vi "Sam_orderfilenames.vi"(9 "Original name":string, 10 "filenames":string[](array[string])) -> (2 "Array 3":cluster{cluster{string[]}[]}[](array[cluster]))   [LabVIEW 2022 SP3]
panel:
  out "Array 2":cluster{string[]}[](array[cluster])
  out "Array":cluster{"Set":string, "Pos":i32, "hit":i32}[](array[cluster])
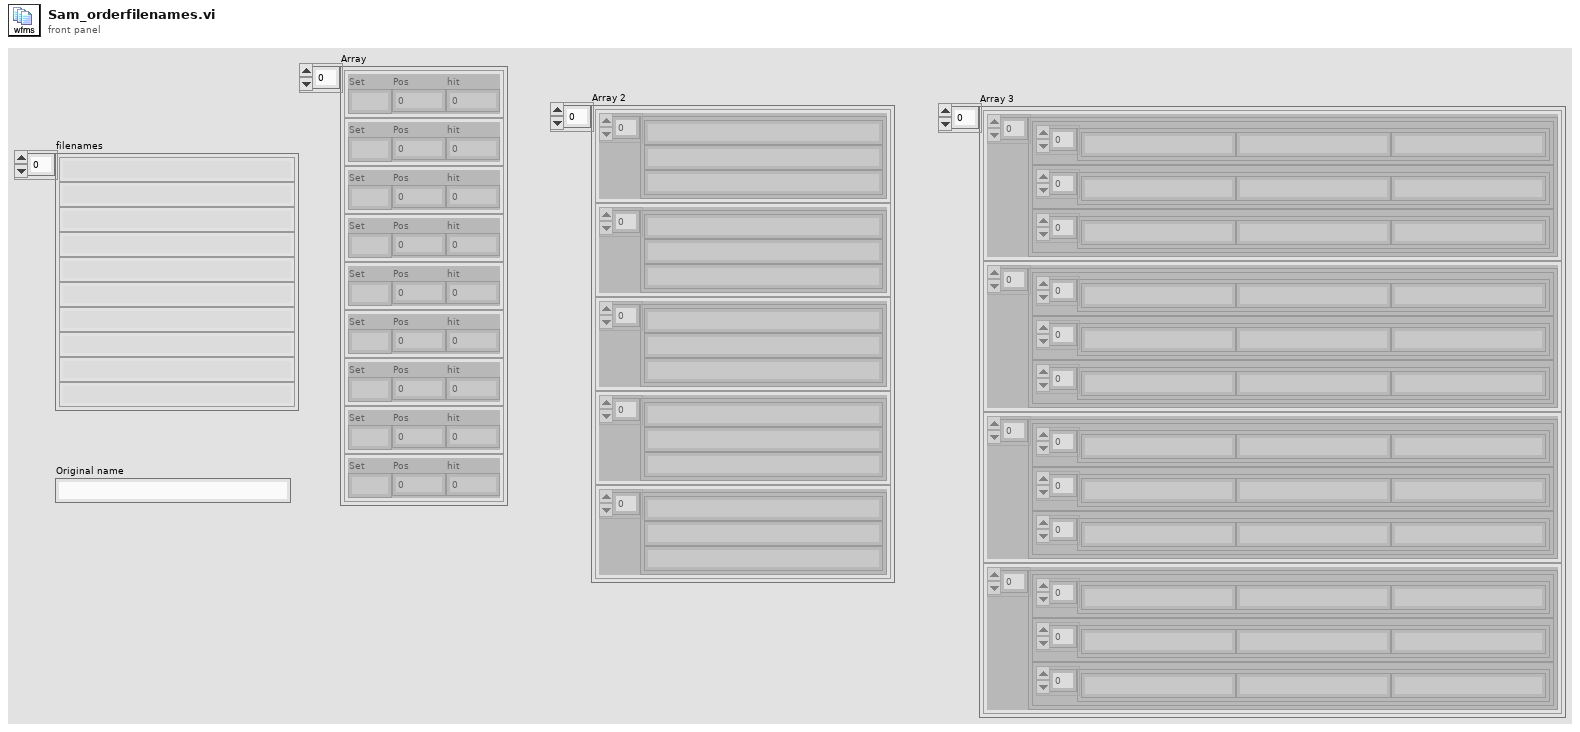
[diagram p1: front panel]
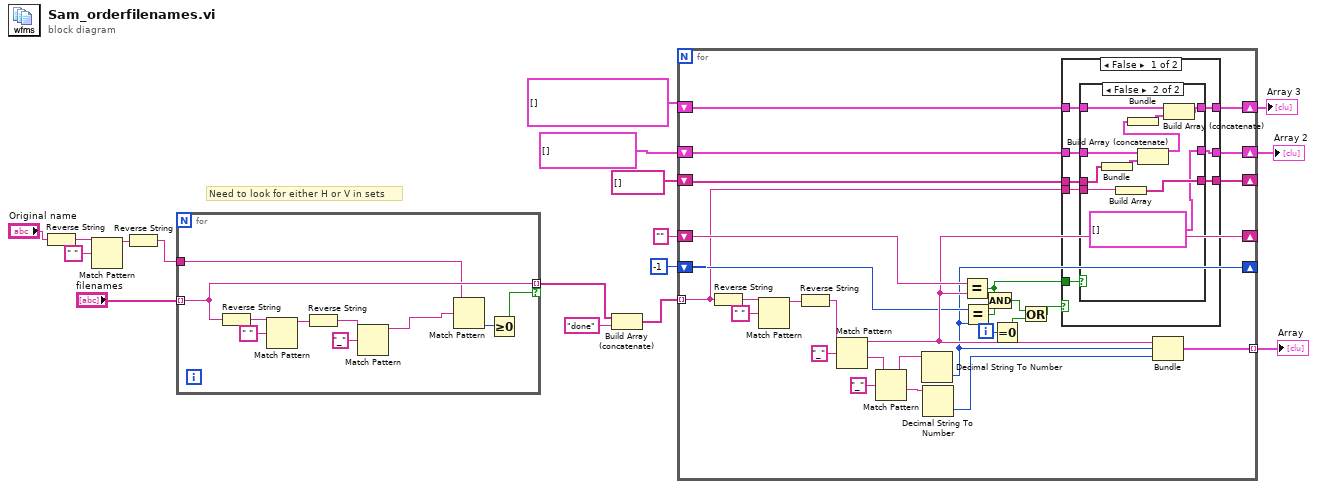
[diagram p0: block diagram]
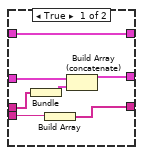
[diagram p2: hidden frame]
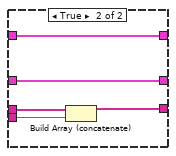
[diagram p3: hidden frame]
diagram:
  # "Need to look for either H or V in sets"
  n1 = Reverse String(1:"Original name") -> (0:w3:string)
  n2 = Match Pattern(string=w3, regular expression=" ") -> (before substring=w5:string)  [unwired: 1 in, 3 out]
  n3 = Reverse String(1:w5) -> (0:w1:string)
  n4 = for {
    tunnel: "filenames" -> [w20] mode=indexing
    tunnel: [w20] -> w6 mode=indexing if=w26
    tunnel: w1 -> [w18]
    n5 = Reverse String(1:w20) -> (0:w25:string)
    n6 = Match Pattern(string=w25, regular expression=" ") -> (before substring=w23:string)  [unwired: 1 in, 3 out]
    n7 = Reverse String(1:w23) -> (0:w21:string)
    n8 = Match Pattern(string=w21, regular expression="_") -> (before substring=w19:string)  [unwired: 1 in, 3 out]
    n9 = Match Pattern(string=w18, regular expression=w19) -> (offset past match=w27:i32)  [unwired: 1 in, 3 out]
    n10 = Greater Or Equal To 0?(x=w27) -> (x >= 0?=w26:bool)
  }
  n11 = Build Array (concatenate)(w6, "done") -> (w9:string[])
  n12 = for {
    tunnel: w9 -> [w39] mode=indexing
    tunnel: [w47] -> w17 mode=indexing
    shift-right: [w43] -> _
    shift-left: "" -> [w44]
    shift-right: [w41] -> _
    shift-left: -1 -> [w42]
    shift-right: [w37] -> _
    shift-left: string[] [] -> [w38]
    shift-right: [w35] -> w8
    shift-left: cluster{string[]}[] [] -> [w36]
    shift-right: [w33] -> w11
    shift-left: cluster{cluster{string[]}[]}[] [] -> [w32]
    i -> [w31]
    n13 = Reverse String(1:w39) -> (0:w55:string)
    n14 = Match Pattern(string=w55, regular expression=" ") -> (before substring=w53:string)  [unwired: 1 in, 3 out]
    n15 = Reverse String(1:w53) -> (0:w51:string)
    n16 = Match Pattern(string=w51, regular expression="_") -> (before substring=w43:string, after substring=w49:string)  [unwired: 1 in, 2 out]
    n17 = Match Pattern(string=w49, regular expression="_") -> (before substring=w48:string, after substring=w46:string)  [unwired: 1 in, 2 out]
    n18 = Decimal String To Number(string=w48) -> (number=w41:i32)  [unwired: 2 in, 1 out]
    n19 = Decimal String To Number(string=w46) -> (number=w45:i32)  [unwired: 2 in, 1 out]
    n20 = Equal?(x=w44, y=w43) -> (x = y?=w34:bool)
    n21 = Equal?(x=w42, y=w41) -> (x = y?=w40:bool)
    n22 = Compound Arithmetic op=AND(w34, w40) -> (w30:bool)
    n23 = Equal To 0?(x=w31) -> (x = 0?=w29:bool)
    n24 = Or(x=w30, y=w29) -> (x .or. y?=w28:bool)
    n25 = case shown="False" w28 {
      tunnel: w39 -> [w63 w85]
      tunnel: w38 -> [w61 w84]
      tunnel: [w62 w83] -> w37
      tunnel: w36 -> [w60 w82]
      tunnel: [w59 w82] -> w35
      tunnel: w34 -> [w58 _]
      tunnel: [w57 w81] -> w33
      tunnel: w32 -> [w56 w81]
      frame False {
        n26 = case shown="False" w58 {
          tunnel: w63 -> [w70 w80]
          tunnel: [w69 w79] -> w62
          tunnel: w61 -> [w68 w78]
          tunnel: w60 -> [w66 w76]
          tunnel: [w65 cluster{string[]}[] []] -> w59
          tunnel: [w64 w73] -> w57
          tunnel: w56 -> [w64 w72]
          frame True {
            n27 = Bundle(w68) -> (w67:cluster{string[]})  [unwired: 1 in]
            n28 = Build Array(w70) -> (w69:string[])
            n29 = Build Array (concatenate)(w66, w67) -> (w65:cluster{string[]}[])
          }
          frame False {
            n30 = Bundle(w78) -> (w77:cluster{string[]})  [unwired: 1 in]
            n31 = Build Array(w80) -> (w79:string[])
            n32 = Build Array (concatenate)(w76, w77) -> (w74:cluster{string[]}[])
            n33 = Bundle(w74) -> (w75:cluster{cluster{string[]}[]})  [unwired: 1 in]
            n34 = Build Array (concatenate)(w72, w75) -> (w73:cluster{cluster{string[]}[]}[])
          }
        }
      }
      frame True {
        n35 = Build Array (concatenate)(w84, w85) -> (w83:string[])
      }
    }
    n36 = Bundle(w43, w41, w45) -> (w47:cluster{string, i32, i32})  [unwired: 1 in]
  }
  "Array" <- w17
  "Array 2" <- w8
  "Array 3" <- w11
